vi "Get Apply Module Mode.vi"(8 "error in (no error)":errorcluster, 11 "Device Item Ref in":T1 format="%.0x") -> (0 "error out":errorcluster, 2 "Apply Module Mode":bool, 3 "Device Item Ref out":T1 format="%.0x")   [LabVIEW 2019, in "SEECD System Explorer.lvlib"]
uses:
  SEECD System Explorer.lvlib
  <vilib>/NI VeriStand/Custom Device Tools/Custom Device Utility Library/Custom Device Utility Library.lvlib
  <vilib>/NI VeriStand/Custom Device Tools/Custom Device Utility Library/NI VeriStand - Search for Item by GUID.vi
  Shared/Globals/Scan Engine GUIDs.vi
  Shared/SEECD Shared.lvlib
  Shared/Globals/Property Strings.vi
  <vilib>/NI VeriStand/Custom Device API/Custom Device API.lvlib
  <vilib>/NI VeriStand/Custom Device API/Custom Device Item Ref.ctl
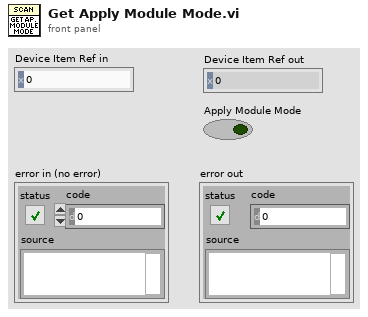
[diagram p1: front panel]
types:
  T1 = typedef "Custom Device API.lvlib/Custom Device Item Ref.ctl" = u64
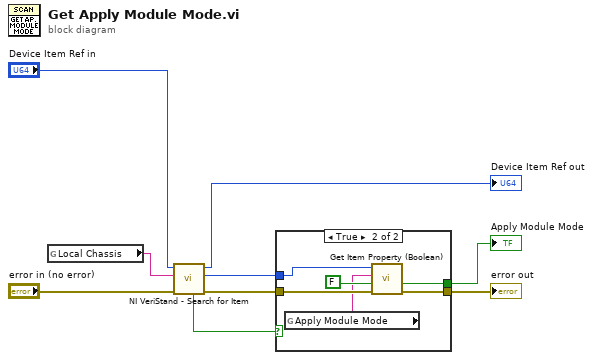
[diagram p0: block diagram]
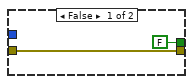
[diagram p2: hidden frame]
diagram:
  n1 = global read "Scan Engine GUIDs.vi" "Local Chassis"() -> (w2:string)
  n2 = call-poly <vilib>:"NI VeriStand - Search for Item.vi"("error in"="error in (no error)", "Item GUID"=w2, "Section Ref in"="Device Item Ref in") -> ("error out"=w5:errorcluster, "Item Ref"=w6:T1, "Section Ref out"=→"Device Item Ref out":T1, "Found"=w4:bool)  [unwired: 5 in]
  n3 = case shown="True" w4 {
    tunnel: w5 -> [w11 w17]
    tunnel: w6 -> [_ w14]
    tunnel: [w11 w13] -> w9
    tunnel: [FALSE ("Value") w12] -> w7
    frame False {
    }
    frame True {
      n4 = global read "Property Strings.vi" "Apply Module Mode"() -> (w15:string)
      n5 = call <vilib>:"Get Item Property (Boolean).vi"("error in (no error)"=w17, "Default Value"=FALSE, "Property Name"=w15, "Item Ref in"=w14) -> ("error out"=w13:errorcluster, "Value"=w12:bool)  [unwired: 4 in, 2 out]
    }
  }
  "error out" <- w9
  "Apply Module Mode" <- w7
